vi "FdxCmdTxStatusCvi.vi"(8 "error in":errorcluster, 11 "InstrumentHandle_port":u32) -> (0 "error out":errorcluster, 1 "TxStatus":T1 {"TransmitMode" items=["FDX_TX_GENERIC", "FDX_TX_REPLAY", "FDX_TX_INDIVIDUAL"]; "TxStatus" items=["FDX_STAT_STOP", "FDX_STAT_RUN", "FDX_STAT_ERROR", "FDX_STAT_WAIT_F_TRIG"]}, 3 "InstrumentHandle_port":u32)   [LabVIEW 2020, in "AIM664LV.lvlib"]
doc: "This function is used to retrieve the transmitter status of the board"
uses:
  AIM664LV.lvlib
  AFDX_LibraryAdmin/FdxGlobalDllPath.vi
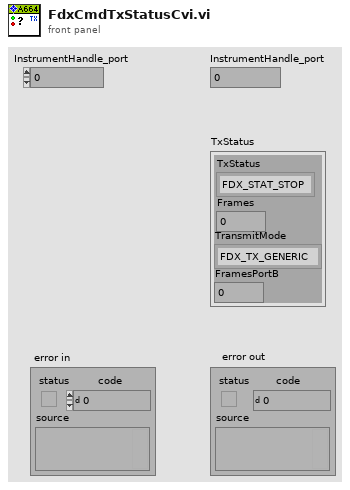
[diagram p1: front panel]
types:
  T1 = cluster{"TxStatus":u32, "Frames":u32, "TransmitMode":u32, "FramesPortB":u32}
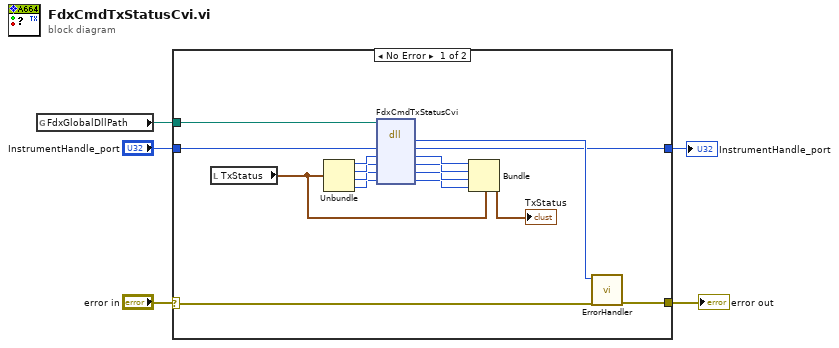
[diagram p0: block diagram]
diagram:
  n1 = global read "FdxGlobalDllPath.vi" "FdxGlobalDllPath"() -> (w3:path)
  n2 = case shown="No Error" "error in" {
    selector: "error in" -> [w20 w23]
    tunnel: [w21 w23] -> w5
    tunnel: w3 -> [w8 _]
    tunnel: "InstrumentHandle_port" -> [w7 w22]
    tunnel: [w6 w22] -> w1
    frame No Error {
      n3 = local read "TxStatus"() -> (w13:T1)
      n4 = Unbundle(w13) -> ("TxStatus"=w12:u32, "Frames"=w11:u32, "TransmitMode"=w10:u32, "FramesPortB"=w9:u32)
      n5 = dll-call lib="aim_fdx.19.dll" fn="FdxCmdTxStatusCvi"(path in=w8, "InstrumentHandle"=w7, "TxStatus"=w12, "Frames"=w11, "TransmitMode"=w10, "FramesPortB"=w9) -> ("status"=w19:i32, "InstrumentHandle"=w6:u32, "TxStatus"=w18:u32, "Frames"=w17:u32, "TransmitMode"=w16:u32, "FramesPortB"=w15:u32)  [unwired: 2 in, 2 out]
      n6 = Bundle(cluster=w13, "TxStatus"=w18, "Frames"=w17, "TransmitMode"=w16, "FramesPortB"=w15) -> (→"TxStatus":T1)
      n7 = call "ErrorHandler.vi"("error in"=w20, "AIM Error"=w19) -> ("error out"=w21:errorcluster)  [unwired: 9 in]
    }
    frame Error {
    }
  }
  "error out" <- w5
  "InstrumentHandle_port" <- w1
